vi "Do.vi"(8 "error in (no error)":errorcluster, 10 "Actor in":refnum<class "Actor.lvclass">, 11 "Device State Information Update Msg":refnum<class "Device State Information Update Msg.lvclass">) -> (0 "error out":errorcluster, 2 "Actor out":refnum<class "Actor.lvclass">)   [LabVIEW 2018, in "EMS User Interface Actor.lvlib" / "Device State Information Update Msg.lvclass"]
doc: "This VI delivers the message to the actor by calling the appropriate method(s) on the actor."
uses:
  Device State Information Update Msg.lvclass
  C:/Users/Administrator/Desktop/2018LabVIEW EMS/EMS Generic Actor/EMS Generic Messages/Device State Information Msg/Device State Information Msg.lvclass
  <vilib>/ActorFramework/Actor/Actor.lvclass
  EMS User Interface/EMS User Interface.lvclass
  C:/Program Files (x86)/National Instruments/LabVIEW 2018/vi.lib/ActorFramework/Actor/Actor.lvclass
  EMS Generic Actor/EMS Generic Messages/Device State Information Msg/Device State Information Msg.lvclass/Device State Information Msg.ctl
  EMS Generic Actor/EMS Generic Messages/Device State Information Msg/Device State Information Msg.lvclass
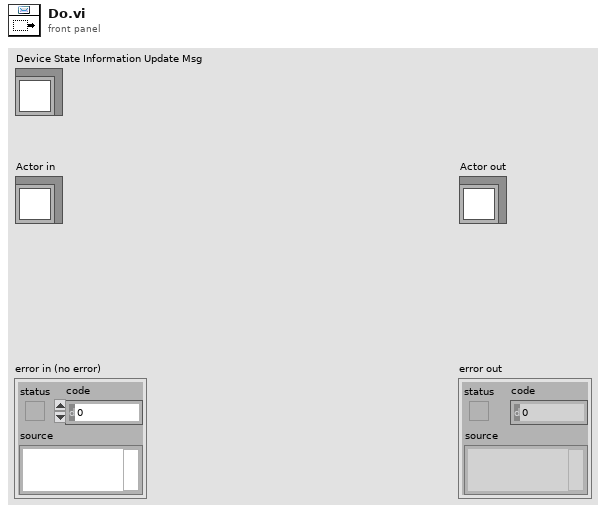
[diagram p1: front panel]
types:
  T1 = typedef "EMS Generic Actor.lvlib/EMS Generic.lvclass/Device Information Cluster.ctl" = cluster{"Device State":T2, "data":variant}
  T2 = typedef "EMS Generic Actor.lvlib/EMS Generic.lvclass/Device State.ctl" = enum16{"Invalid", "Clear", "DevIDs in Config", "DevIDs on uGrid", "DevIDs not on uGrid", "Update IED_Status", "Update DER_Status", "Update DER_Measurement", "Update SmartRelay_Measurement"}
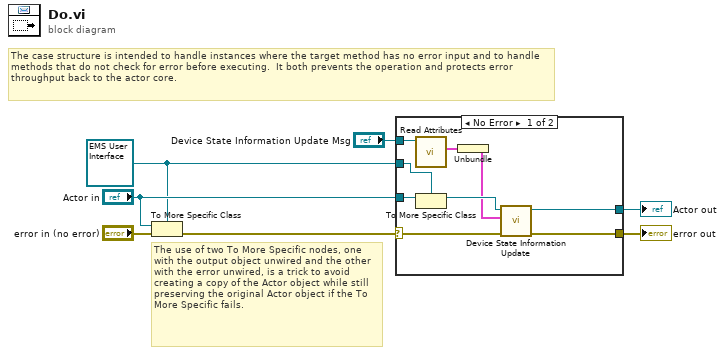
[diagram p0: block diagram]
diagram:
  w2 = refnum<class "EMS User Interface.lvclass"> refnum ("Actor in")
  # "The use of two To More Specific nodes, one with the output object unwired and the other with the error unwired, is a trick to avoid creating a copy of the Actor object while still preserving the original Actor object if the To More Specific fails."
  # "The case structure is intended to handle instances where the target method has no error input and to handle methods that do not check for error before executing.  It both prevents the operation and protects error throughput back to the actor core."
  n1 = To More Specific Class(target class=w2, reference="Actor in", error in="error in (no error)") -> (error out=w6:errorcluster)  [unwired: 1 out]
  n2 = case shown="No Error" w6 {
    selector: w6 -> [w14 w18]
    tunnel: [w16 w18] -> w5
    tunnel: [w15 w17] -> w4
    tunnel: "Actor in" -> [w13 w17]
    tunnel: w2 -> [w12 _]
    tunnel: "Device State Information Update Msg" -> [w9 _]
    frame No Error {
      n3 = call "Read Attributes.vi"("Device State Information Msg"=w9) -> ("Payload"=w10:cluster{"Device State Information":T1})  [unwired: 10 in]
      n4 = To More Specific Class(target class=w12, reference=w13) -> (specific class reference=w11:refnum<class "EMS User Interface.lvclass">)  [unwired: 1 in, 1 out]
      n5 = Unbundle(w10) -> ("Device State Information"=w8:T1)
      n6 = call "Device State Information Update.vi"("error in"=w14, "Device State Information"=w8, "EMS User Interface in"=w11) -> ("error out"=w16:errorcluster, "dup EMS User Interface"=w15:refnum<class "EMS User Interface.lvclass">)  [unwired: 7 in]
    }
    frame Error {
      # "If type check fails, pass the original object out again."
    }
  }
  "error out" <- w5
  "Actor out" <- w4
